vi "Teleop Shooter Control.vi"(8 "Driver Axes":T1, 9 "Driver Buttons":T4, 10 "Manipulator Axes":T1, 11 "Manipulator Buttons":T4) -> (3 "Shooter Control":T2)   [LabVIEW 2013]
uses:
  <vilib>/Rock Robotics/WPI/Joystick/WPI_JoystickButtonState.ctl
  Shooter Manual Control.ctl
  Shooter Command.ctl
  Common Code/Change Detect.vi
  Common Code/Change Detect Boolean.vi
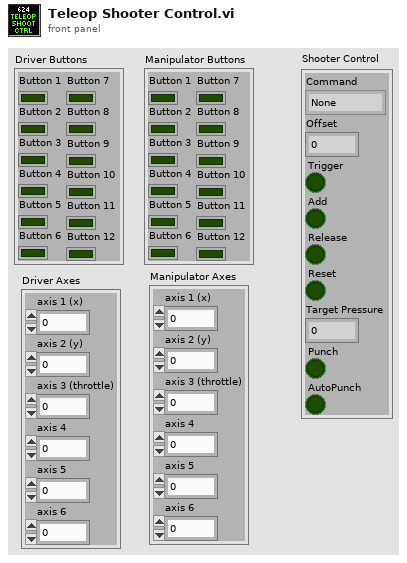
[diagram p1: front panel]
types:
  T1 = cluster{"axis 1 (x)":dbl, "axis 2 (y)":dbl, "axis 3 (throttle)":dbl, "axis 4":dbl, "axis 5":dbl, "axis 6":dbl}
  T2 = typedef "Shooter Manual Control.ctl" = cluster{"Command":T3, "Offset":dbl, "Trigger":bool, "Add":bool, "Release":bool, "Reset":bool, "Target Pressure":dbl, "Punch":bool, "AutoPunch":bool}
  T3 = typedef "Shooter Command.ctl" = enum16{"None", "Warmup", "Shoot", "Line Shoot", "Soft Shoot", "Toss"}
  T4 = typedef "WPI_JoystickButtonState.ctl" = cluster{"Button 1":bool, "Button 2":bool, "Button 3":bool, "Button 4":bool, "Button 5":bool, "Button 6":bool, "Button 7":bool, "Button 8":bool, "Button 9":bool, "Button 10":bool, "Button 11":bool, "Button 12":bool}
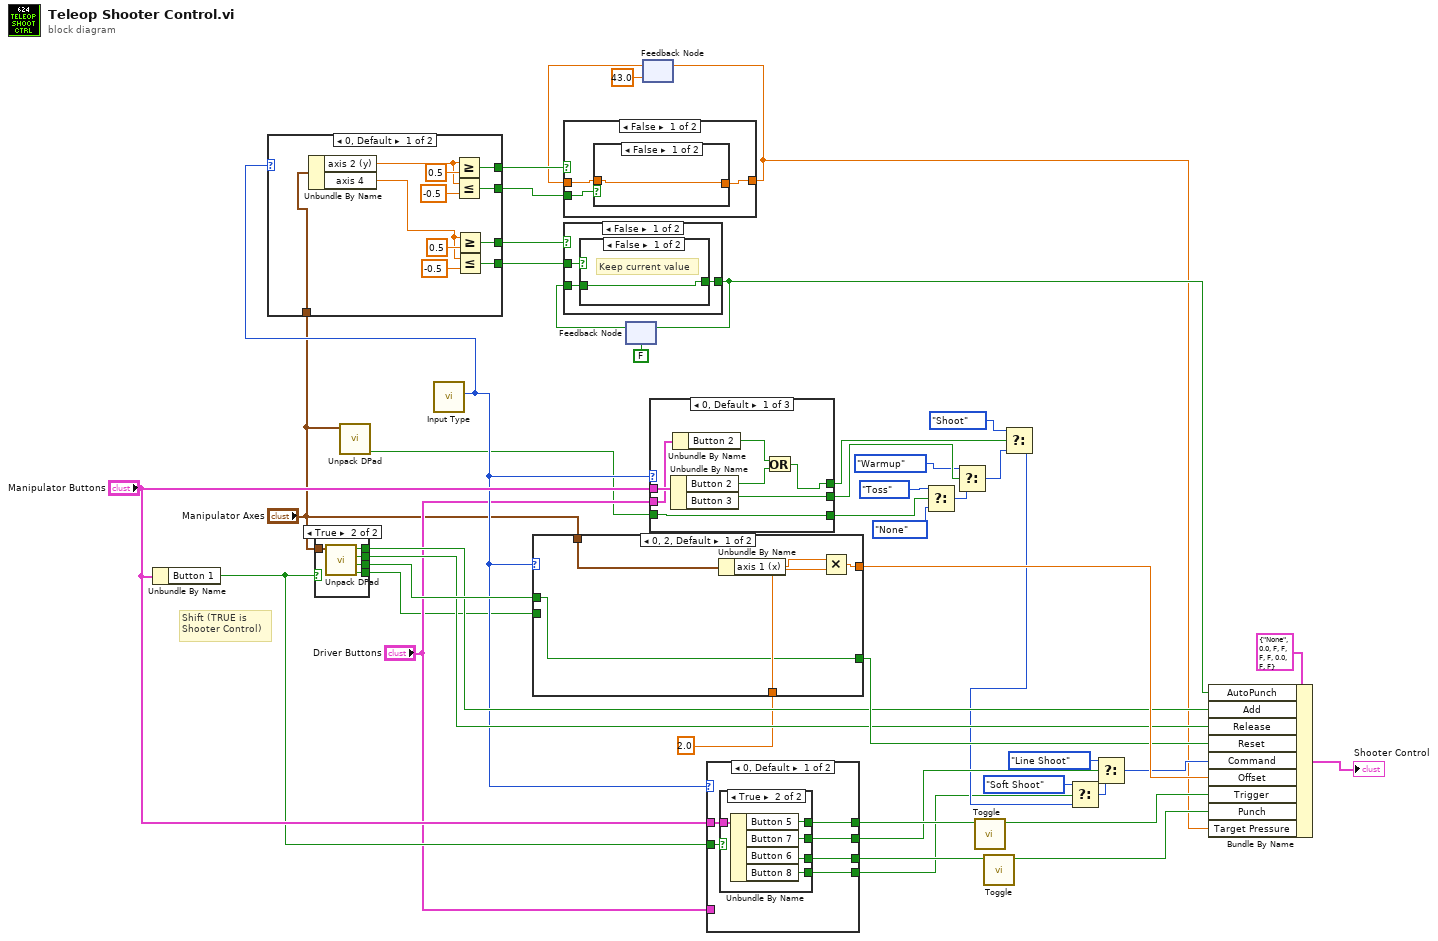
[diagram p0: block diagram]
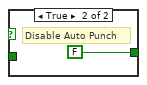
[diagram p2: hidden frame]
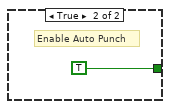
[diagram p3: hidden frame]
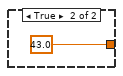
[diagram p4: hidden frame]
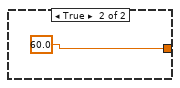
[diagram p5: hidden frame]
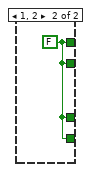
[diagram p6: hidden frame]
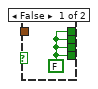
[diagram p7: hidden frame]
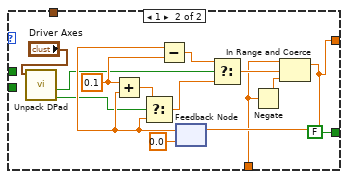
[diagram p8: hidden frame]
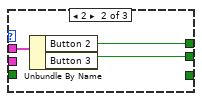
[diagram p9: hidden frame]
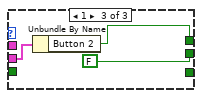
[diagram p10: hidden frame]
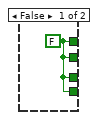
[diagram p11: hidden frame]
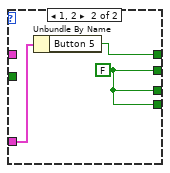
[diagram p12: hidden frame]
diagram:
  # "Shift (TRUE is\nShooter Control)"
  n1 = Unbundle By Name("Manipulator Buttons") -> ("Button 1"=w31:bool)
  n2 = case shown="True" w31 {
    tunnel: [w46 w51] -> w4
    tunnel: [w46 w50] -> w36
    tunnel: [w46 w49] -> w35
    tunnel: [w46 w48] -> w34
    tunnel: "Manipulator Axes" -> [_ w47]
    frame False {
      w46 = FALSE
    }
    frame True {
      n3 = call "Unpack DPad.vi"("Axes"=w47) -> ("Right"=w51:bool, "Left"=w50:bool, "Down"=w49:bool, "Up"=w48:bool)  [unwired: 7 in]
    }
  }
  n4 = call "Unpack DPad.vi"("Axes"="Manipulator Axes") -> ("Right"=w1:bool)  [unwired: 7 in, 3 out]
  n5 = call "Input Type.vi"() -> ("Mode"=w25:i32)  [unwired: 11 in]
  n6 = case shown="0, Default" w25 {
    tunnel: "Manipulator Axes" -> [w57 _]
    tunnel: [w59 w63] -> w24
    tunnel: [w58 w63] -> w23
    tunnel: [w53 w63] -> w22
    tunnel: [w52 w63] -> w21
    frame 0, Default {
      n7 = Unbundle By Name(w57) -> ("axis 2 (y)"=w60:dbl, "axis 4"=w54:dbl)
      n8 = Greater Or Equal?(x=w60, y=0.5) -> (x >= y?=w58:bool)
      n9 = Less Or Equal?(x=w60, y=-0.5) -> (x <= y?=w59:bool)
      n10 = Greater Or Equal?(x=w54, y=0.5) -> (x >= y?=w53:bool)
      n11 = Less Or Equal?(x=w54, y=-0.5) -> (x <= y?=w52:bool)
    }
    frame 1, 2 {
      w63 = FALSE
    }
  }
  n12 = case shown="0, 2, Default" w25 {
    tunnel: 2.0 -> [w67 w73]
    tunnel: [w66 w74] -> w43
    tunnel: w36 -> [w65 _]
    tunnel: [w65 FALSE ("Left")] -> w41
    tunnel: "Manipulator Axes" -> [w64 _]
    tunnel: w4 -> [_ _]
    frame 0, 2, Default {
      n13 = Unbundle By Name(w64) -> ("axis 1 (x)"=w68:dbl)
      n14 = Multiply(x=w68, y=w67) -> (x*y=w66:dbl)
    }
    frame 1 {
      w77 = 0.1 ("x")
      n15 = call "Unpack DPad.vi"("Axes"="Driver Axes") -> ("Right"=w70:bool, "Left"=w71:bool)  [unwired: 7 in, 2 out]
      n16 = feedback #1(0.0) -> (w78:dbl)
      n17 = Add(x=w77, y=w78) -> (x+y=w79:dbl)
      n18 = Select(t=w79, s=w70, f=w78) -> (s? t:f=w80:dbl)
      n19 = Subtract(x=w78, y=w77) -> (x-y=w81:dbl)
      n20 = Select(t=w81, s=w71, f=w80) -> (s? t:f=w75:dbl)
      n21 = Negate(x=w73) -> (-x=w72:dbl)
      n22 = In Range and Coerce(upper limit=w73, x=w75, lower limit=w72) -> (coerced(x)=w74:dbl)  [unwired: 1 out]
      n23 = feedback-in #1(w74) -> ()
    }
  }
  n24 = feedback #2(FALSE) -> (w19:bool)
  n25 = case shown="False" w22 {
    tunnel: w21 -> [w85 _]
    tunnel: w19 -> [w83 _]
    tunnel: [w84 TRUE] -> w18
    frame False {
      n26 = case shown="False" w85 {
        tunnel: [w86 FALSE] -> w84
        tunnel: w83 -> [w86 _]
        frame False {
          # "Keep current value"
        }
        frame True {
          # "Disable Auto Punch"
        }
      }
    }
    frame True {
      # "Enable Auto Punch"
    }
  }
  n27 = feedback-in #2(w18) -> ()
  n28 = feedback #3(43.0 ("Numeric")) -> (w15:dbl)
  n29 = case shown="False" w23 {
    tunnel: w24 -> [w91 _]
    tunnel: [w90 60.0 ("Numeric")] -> w13
    tunnel: w15 -> [w89 _]
    frame False {
      n30 = case shown="False" w91 {
        tunnel: [w92 43.0 ("Numeric")] -> w90
        tunnel: w89 -> [w92 _]
        frame False {
        }
        frame True {
        }
      }
    }
    frame True {
    }
  }
  n31 = feedback-in #3(w13) -> ()
  n32 = case shown="0, Default" w25 {
    tunnel: "Manipulator Buttons" -> [w101 w104 _]
    tunnel: [w100 w103 FALSE ("Button 3")] -> w45
    tunnel: [w96 w102 w107] -> w16
    tunnel: "Driver Buttons" -> [w99 _ w105]
    tunnel: w1 -> [w95 _ _]
    tunnel: [w95 _ _] -> w3
    frame 0, Default {
      n33 = Unbundle By Name(w101) -> ("Button 2"=w97:bool, "Button 3"=w100:bool)
      n34 = Unbundle By Name(w99) -> ("Button 2"=w98:bool)
      n35 = Or(x=w98, y=w97) -> (x .or. y?=w96:bool)
    }
    frame 2 {
      n36 = Unbundle By Name(w104) -> ("Button 2"=w102:bool, "Button 3"=w103:bool)
    }
    frame 1 {
      n37 = Unbundle By Name(w105) -> ("Button 2"=w107:bool)
    }
  }
  n38 = case shown="0, Default" w25 {
    tunnel: "Driver Buttons" -> [_ w122]
    tunnel: [w113 w121] -> w38
    tunnel: "Manipulator Buttons" -> [w112 _]
    tunnel: w31 -> [w111 _]
    tunnel: [w108 w120] -> w28
    tunnel: [w110 w120] -> w26
    tunnel: [w109 w120] -> w9
    frame 0, Default {
      n39 = case shown="True" w111 {
        tunnel: [w114 w119] -> w113
        tunnel: w112 -> [_ w118]
        tunnel: [w114 w117] -> w108
        tunnel: [w114 w116] -> w110
        tunnel: [w114 w115] -> w109
        frame False {
          w114 = FALSE ("Button 5")
        }
        frame True {
          n40 = Unbundle By Name(w118) -> ("Button 5"=w119:bool, "Button 7"=w117:bool, "Button 6"=w116:bool, "Button 8"=w115:bool)
        }
      }
    }
    frame 1, 2 {
      w120 = FALSE ("Button 7")
      n41 = Unbundle By Name(w122) -> ("Button 5"=w121:bool)
    }
  }
  n42 = Select(t=Shooter_Command."Toss", s=w3, f=Shooter_Command."None" ("Shoot Command")) -> (s? t:f=w7:T3)
  n43 = Select(t=Shooter_Command."Warmup" ("Shoot Command"), s=w45, f=w7) -> (s? t:f=w44:T3)
  n44 = call "Toggle.vi"("In"=w38) -> ("Toggled"=w37:bool)  [unwired: 10 in]
  n45 = call "Toggle.vi"("In"=w26) -> ("Toggled"=w27:bool)  [unwired: 10 in]
  n46 = Select(t=Shooter_Command."Shoot" ("Shoot Command"), s=w16, f=w44) -> (s? t:f=w11:T3)
  n47 = Select(t=Shooter_Command."Soft Shoot" ("Shoot Command"), s=w9, f=w11) -> (s? t:f=w8:T3)
  n48 = Select(t=Shooter_Command."Line Shoot" ("Shoot Command"), s=w28, f=w8) -> (s? t:f=w29:T3)
  n49 = Bundle By Name(cluster=T2 {"Command"=enum."None", "Offset"=0.0, "Trigger"=FALSE, "Add"=FALSE, "Release"=FALSE, "Reset"=FALSE, "Target Pressure"=0.0, "Punch"=FALSE, "AutoPunch"=FALSE} ("Shooter Manual Control"), "AutoPunch"=w18, "Add"=w34, "Release"=w35, "Reset"=w41, "Command"=w29, "Offset"=w43, "Trigger"=w37, "Punch"=w27, "Target Pressure"=w13) -> (→"Shooter Control":T2)
